vi "Waveform_shift.vi"(10 "Waveform_in":waveform(dbl)) -> (2 "Peak Value":dbl)   [LabVIEW 2019]
uses:
  SiPM_Tests_Global_Var.vi
  <vilib>/Analysis/NI_AALPro.lvlib
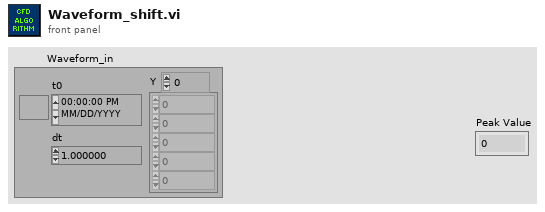
[diagram p1: front panel]
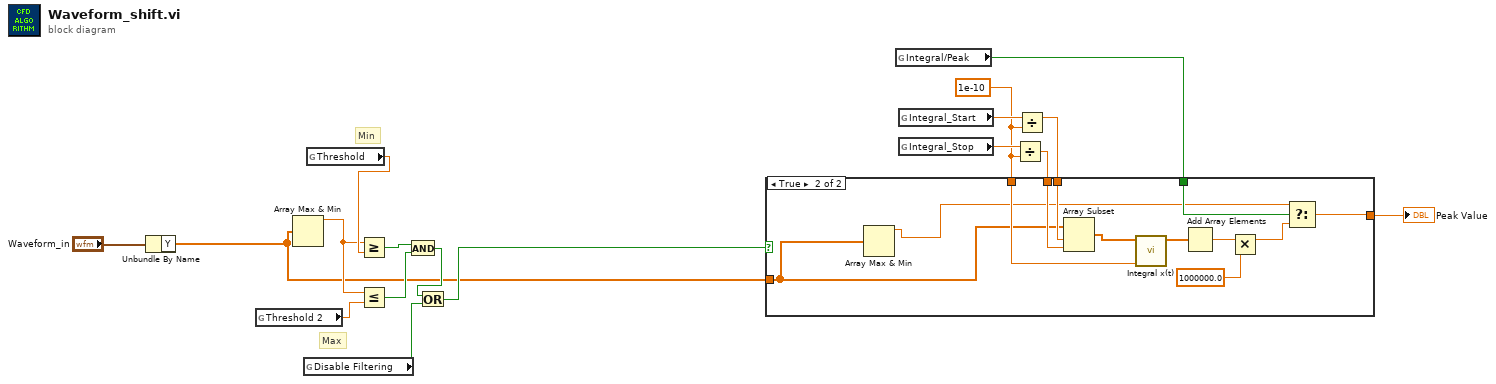
[diagram p0: block diagram]
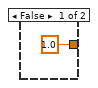
[diagram p2: hidden frame]
diagram:
  w3 = 1e-10 ("dt")
  # "Max"
  # "Min"
  n1 = Unbundle By Name("Waveform_in") -> ("Y"=w1:dbl[])
  n2 = global read "SiPM_Tests_Global_Var.vi" "Threshold 2"() -> (w13:dbl)
  n3 = Array Max & Min(array=w1) -> (max value=w14:dbl)  [unwired: 3 out]
  n4 = global read "SiPM_Tests_Global_Var.vi" "Disable Filtering"() -> (w8:bool)
  n5 = global read "SiPM_Tests_Global_Var.vi" "Threshold"() -> (w16:dbl)
  n6 = Greater Or Equal?(x=w14, y=w16) -> (x >= y?=w12:bool)
  n7 = Less Or Equal?(x=w14, y=w13) -> (x <= y?=w11:bool)
  n8 = And(x=w12, y=w11) -> (x .and. y?=w10:bool)
  n9 = Or(x=w10, y=w8) -> (x .or. y?=w9:bool)
  n10 = global read "SiPM_Tests_Global_Var.vi" "Integral/Peak"() -> (w2:bool)
  n11 = global read "SiPM_Tests_Global_Var.vi" "Integral_Start"() -> (w7:dbl)
  n12 = global read "SiPM_Tests_Global_Var.vi" "Integral_Stop"() -> (w6:dbl)
  n13 = Divide(x=w6, y=w3) -> (x/y=w4:dbl)
  n14 = Divide(x=w7, y=w3) -> (x/y=w5:dbl)
  n15 = case shown="True" w9 {
    tunnel: w1 -> [_ w19]
    tunnel: [1.0 w25] -> w15
    tunnel: w5 -> [_ w30]
    tunnel: w4 -> [_ w29]
    tunnel: w3 -> [_ w27]
    tunnel: w2 -> [_ w23]
    frame False {
    }
    frame True {
      n16 = Array Max & Min(array=w19) -> (max value=w20:dbl)  [unwired: 3 out]
      n17 = Array Subset(array=w19, index=w30, length=w29) -> (w28:dbl[])
      n18 = call <vilib>:"Integral x(t).vi"("dt"=w27, "X"=w28) -> ("Integral X"=w26:dbl[])  [unwired: 8 in, 1 out]
      n19 = Add Array Elements(numeric array=w26) -> (sum=w24:dbl)
      n20 = Multiply(x=w24, y=1000000.0) -> (x*y=w22:dbl)
      n21 = Select(t=w20, s=w23, f=w22) -> (s? t:f=w25:dbl)
    }
  }
  "Peak Value" <- w15
